vi "SRV_Append Filepath Extension if Necessary.vi"(5 "Filepath":path, 9 "Extension":string) -> (8 "Filepath with Extension":path)   [LabVIEW 2014]
doc: "Appends Extension to the filename in Filepath if the specified extension is not already the end of filename.\n\n\nAuthor: Mike Schultz"
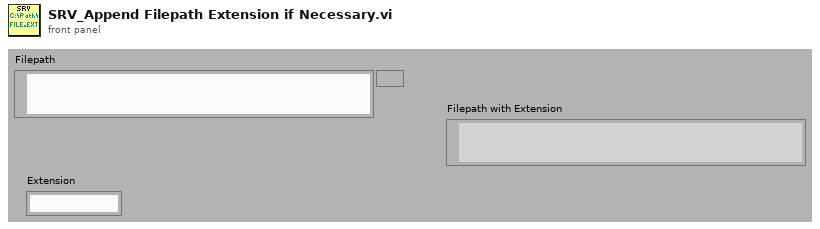
[diagram p1: front panel]
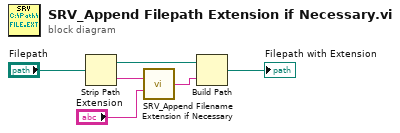
[diagram p0: block diagram]
diagram:
  n1 = Strip Path(path="Filepath") -> (stripped path=w2:path, name=w5:string)
  n2 = call "SRV_Append Filename Extension if Necessary.vi"("Filename"=w5, "Extension"="Extension") -> ("Filename with Extension"=w3:string)  [unwired: 13 in]
  n3 = Build Path(base path=w2, name or relative path=w3) -> (appended path=→"Filepath with Extension":path)
